vi "Validate Instrument Addon Name Is Not In Use.vi"(8 "Error In":errorcluster, 10 "Name In":string, 11 "Instrument Addon Refnum In":T1 format="%.0x") -> (0 "Error Out":errorcluster, 2 "Name Out":string, 3 "Instrument Addon Refnum Out":T1=18446744073709551615 format="%.0x")   [LabVIEW 2023, in "Instrument Addon Scripting API.lvlib"]
doc: "Verifies if the desired name is already in use by a different Instrument Addon Custom Device.\n\nInput: \nInstrument Addon Refnum In: represents the reference to the Instrument Addon Custom Device\nName In: represents the desired name for the Custom Device\n\nOutput:\nInstrument Addon Refnum Our: represents the reference to the Instrument Addon Custom Device provided as input\nName Out: represents the desired name provided as input"
uses:
  Instrument Addon Scripting API.lvlib
  <vilib>/NI VeriStand/Custom Device API/Custom Device Item Ref.ctl
  Addon/Addon Shared/SubVIs/Constants.vi
  <vilib>/NI/NI VeriStand Advanced SysDef API/_SubVIs/SysDef.Search.GUIDs.vi
  NationalInstruments.VeriStand.SystemDefinitionAPI
  <vilib>/NI/NI VeriStand Advanced SysDef API/SysDef API/Advanced System Definition.lvlib
  Addon/Addon Shared/Instrument Addon Shared.lvlib
  <vilib>/NI VeriStand/Custom Device API/Custom Device API.lvlib
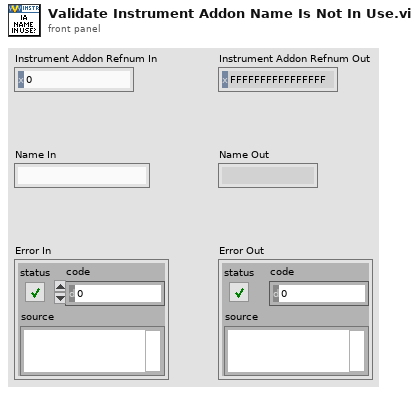
[diagram p1: front panel]
types:
  T1 = typedef "Custom Device API.lvlib/Custom Device Item Ref.ctl" = u64
  T2 = typedef "Advanced System Definition.lvlib/TreeItem.Info.ctl" = cluster{"Name":string, "Description":string, "GUID":string, "Is Channel":bool, "Channel":T3, "Is Waveform":bool, "Waveform":T5}
  T3 = typedef "Custom Device API.lvlib/Custom Device Channel.ctl" = cluster{"Type":T4, "Units":string, "Default Value":dbl, "Faultable":bool, "Scalable":bool}
  T4 = typedef "Custom Device API.lvlib/Custom Device Channel Type.ctl" = enum16{"Input", "Output"}
  T5 = typedef "Custom Device API.lvlib/Custom Device Waveform.ctl" = cluster{"Data Type":T6, "Units":string}
  T6 = typedef "Custom Device API.lvlib/Custom Device Waveform DataType.ctl" = enum16{"Double", "Complex Double"}
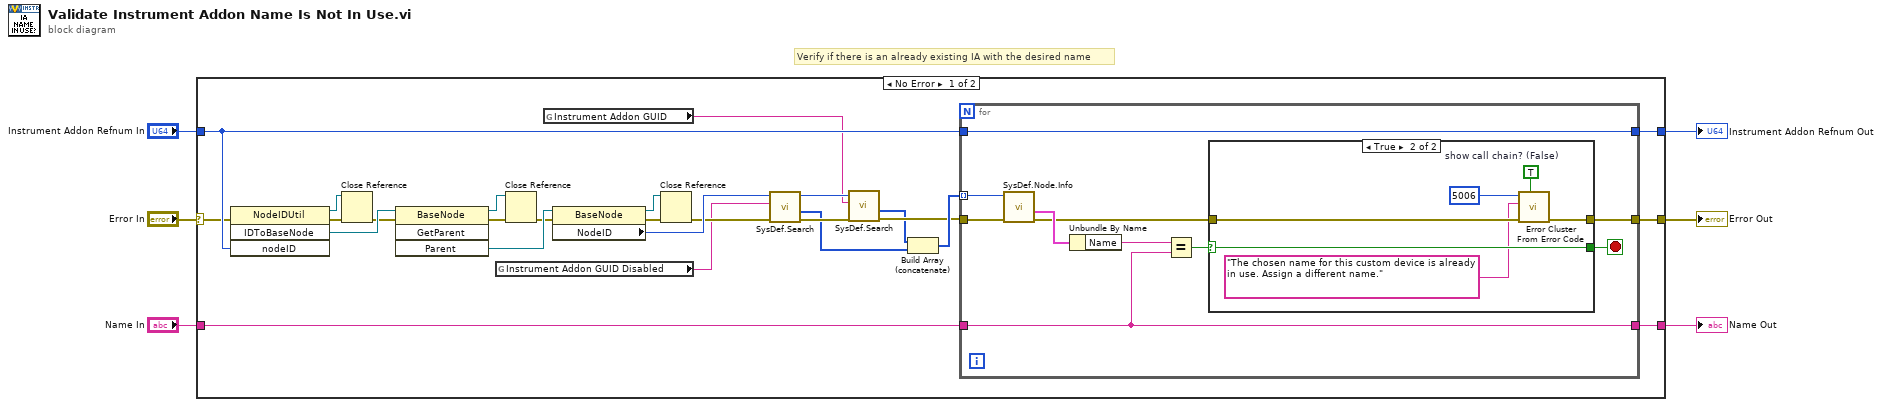
[diagram p0: block diagram]
diagram:
  # "Verify if there is an already existing IA with the desired name"
  n1 = case shown="No Error" "Error In" {
    selector: "Error In" -> [w15 w52]
    tunnel: "Name In" -> [w29 w51]
    tunnel: [w28 w52] -> w5
    tunnel: [w27 w51] -> w4
    tunnel: "Instrument Addon Refnum In" -> [w26 w53]
    tunnel: [w25 w53] -> w2
    frame No Error {
      n2 = invoke class="NodeIDUtil" method="IDToBaseNode"(error in=w15, "nodeID"=w26) -> (reference out=w22:refnum<k24>, error out=w24:errorcluster, "IDToBaseNode"=w32:refnum<k24>)  [unwired: 2 in, 1 out]
      n3 = Close Reference(reference=w22, error in (no error)=w24) -> (error out=w23:errorcluster)
      n4 = invoke class="BaseNode" method="GetParent"(reference=w32, error in=w23) -> (reference out=w20:refnum<k24>, error out=w21:errorcluster, "Parent"=w31:refnum<k24>)  [unwired: 2 in, 1 out]
      n5 = global read "Constants.vi" "Instrument Addon GUID Disabled"() -> (w10:string)
      n6 = Close Reference(reference=w20, error in (no error)=w21) -> (error out=w19:errorcluster)
      n7 = global read "Constants.vi" "Instrument Addon GUID"() -> (w7:string)
      n8 = property class="BaseNode"(reference=w31, error in=w19) -> (reference out=w17:refnum<k24>, error out=w18:errorcluster, "NodeID"=w30:u64)
      n9 = Close Reference(reference=w17, error in (no error)=w18) -> (error out=w16:errorcluster)
      n10 = call-poly <vilib>:"SysDef.Search.vi"("error in (no error)"=w16, "GUID"=w10, "nodeID"=w30) -> ("error out"=w14:errorcluster, "Values Out"=w9:u64[], "nodeID out"=w13:u64)  [unwired: 5 in, 1 out]
      n11 = call-poly <vilib>:"SysDef.Search.vi"("error in (no error)"=w14, "GUID"=w7, "nodeID"=w13) -> ("error out"=w11:errorcluster, "Values Out"=w8:u64[])  [unwired: 5 in, 2 out]
      n12 = Build Array (concatenate)(w8, w9) -> (w12:u64[])
      n13 = for {
        tunnel: w29 -> [w35]
        tunnel: w11 -> [w42]
        tunnel: [w36] -> w28
        tunnel: [w35] -> w27
        tunnel: w26 -> [w34]
        tunnel: [w34] -> w25
        tunnel: w12 -> [w33] mode=indexing
        stop <- w37 stop-if-true
        n14 = call <vilib>:"SysDef.Node.Info.vi"("error in (no error)"=w42, "nodeID"=w33) -> ("error out"=w38:errorcluster, "Item Info"=w41:T2)  [unwired: 6 in, 2 out]
        n15 = Unbundle By Name(w41) -> ("Name"=w40:string)
        n16 = Equal?(x=w40, y=w35) -> (x = y?=w39:bool)
        n17 = case shown="True" w39 {
          selector: w39 -> [w43 w50]
          tunnel: w38 -> [w44 w48]
          tunnel: [w43 w50] -> w37
          tunnel: [w44 w49] -> w36
          frame False {
          }
          frame True {
            w45 = TRUE  # show call chain? (False)
            n18 = call <vilib>:"Error Cluster From Error Code.vi"("show call chain? (False)"=w45, "error in (no error)"=w48, "error message (\"\")"="The chosen name for this custom device is already in use. Assign a different name." ("error message (\"\")"), "error code (0)"=5006) -> ("error out"=w49:errorcluster)  [unwired: 5 in]
          }
        }
      }
    }
    frame Error {
    }
  }
  "Error Out" <- w5
  "Name Out" <- w4
  "Instrument Addon Refnum Out" <- w2
